vi "PWM_주기 점유율 제어.vi"() -> ()   [LabVIEW 2014]
uses:
  <vilib>/DAQmx/create/channels.llb/DAQmx Create Channel (CO-Pulse Generation-Frequency).vi
  <vilib>/DAQmx/configure/timing.llb/DAQmx Timing (Implicit).vi
  <vilib>/DAQmx/write.llb/DAQmx Write (Counter Frequency 1Chan 1Samp).vi
panel:
  out "이전 값":dbl
  in  "정지":bool
  in  "counter":tag="cDAQ3Mod1/ctr0" caption="카운터"
  in  "duty cycle":dbl(knob)=0.5 caption="주기 점유율" scale=0.05..0.15
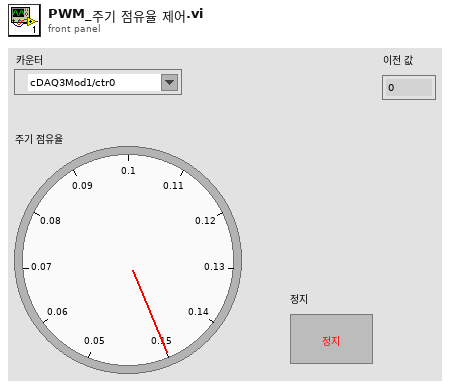
[diagram p1: front panel]
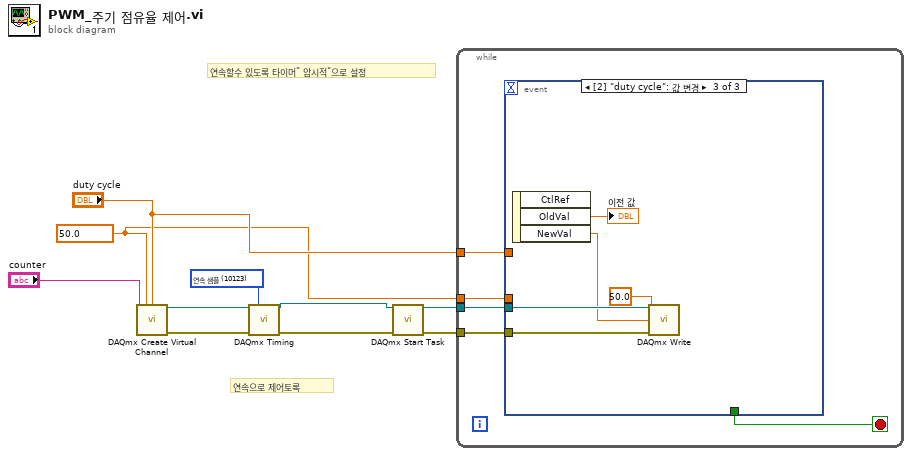
[diagram p0: block diagram]
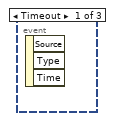
[diagram p2: hidden frame]
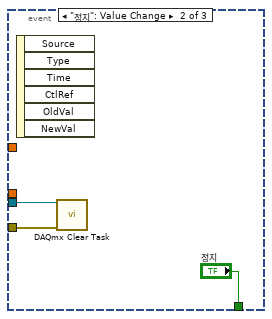
[diagram p3: hidden frame]
diagram:
  w8 = 10123 items=["유한 샘플"=10178, "연속 샘플"=10123, "하드웨어 타이밍에 의한 단일 포인트"=12522] ("sample mode")
  w1 = 50.0 ("frequency")
  # "연속으로 제어토록"
  # "연속할수 있도록 타이머\" 암시적\"으로 설정"
  n1 = call-poly <vilib>:"DAQmx Create Virtual Channel.vi"("frequency"=w1, "duty cycle"="duty cycle", "counter"="counter") -> ("task out"=w9:refnum<k21>, "error out"=w6:errorcluster)  [unwired: 11 in]
  n2 = call-poly <vilib>:"DAQmx Timing.vi"("task/channels in"=w9, "sample mode"=w8, "error in"=w6) -> ("task out"=w7:refnum<k21>, "error out"=w5:errorcluster)  [unwired: 11 in]
  n3 = call <vilib>:"DAQmx Start Task.vi"("task/channels in"=w7, "error in"=w5) -> ("task out"=w4:refnum<k21>, "error out"=w3:errorcluster)  [unwired: 12 in]
  n4 = while {
    tunnel: w4 -> [w15]
    tunnel: w3 -> [w14]
    tunnel: "duty cycle" -> [w12]
    tunnel: w1 -> [w11]
    stop <- w13 stop-if-true
    n5 = event shown="[2] \"duty cycle\": 값 변경" {
      selector: _ -> [_ _ _]
      dyn-events: _ -> [_ _ _]
      timeout: _ -> [_ _ _]
      tunnel: w15 -> [_ w18 w23]
      tunnel: w14 -> [_ w17 w22]
      tunnel: [_ "정지" _] -> w13
      tunnel: w12 -> [_ _ _]
      tunnel: w11 -> [_ _ _]
      event Timeout {
        n6 = event-data() -> ()  [unwired: 1 in, 3 out]
      }
      event "정지": Value Change {
        n7 = event-data() -> ()  [unwired: 1 in, 6 out]
        n8 = call <vilib>:"DAQmx Clear Task.vi"("task in"=w18, "error in"=w17) -> ()  [unwired: 13 in, 1 out]
      }
      event "duty cycle": Value Change {
        n9 = event-data() -> ("OldVal"=→"이전 값":dbl, "NewVal"=w21:dbl)  [unwired: 1 in, 1 out]
        n10 = call-poly <vilib>:"DAQmx Write.vi"("task/channels in"=w23, "frequency"=50.0, "duty cycle"=w21, "error in"=w22) -> ()  [unwired: 9 in, 3 out]
      }
    }
  }
